vi "NewArray2.vi"(6 "Function":enum16{"Default", "Split to new"}(ring)=enum."Split to new", 7 "Map ref":refnum<vi>, 8 "error in (no error)":errorcluster, 11 "All Lines":T1) -> (0 "error out":errorcluster, 3 "output array":T1)   [LabVIEW 2014]
uses:
  Libraries/Map Data Folder/All-Lines.ctl
  Libraries/Map Data Folder/LineCluster.ctl
  Libraries/Map Data Folder/LineConnection.ctl
  Libraries/Map Data Folder/Map Data.lvlib
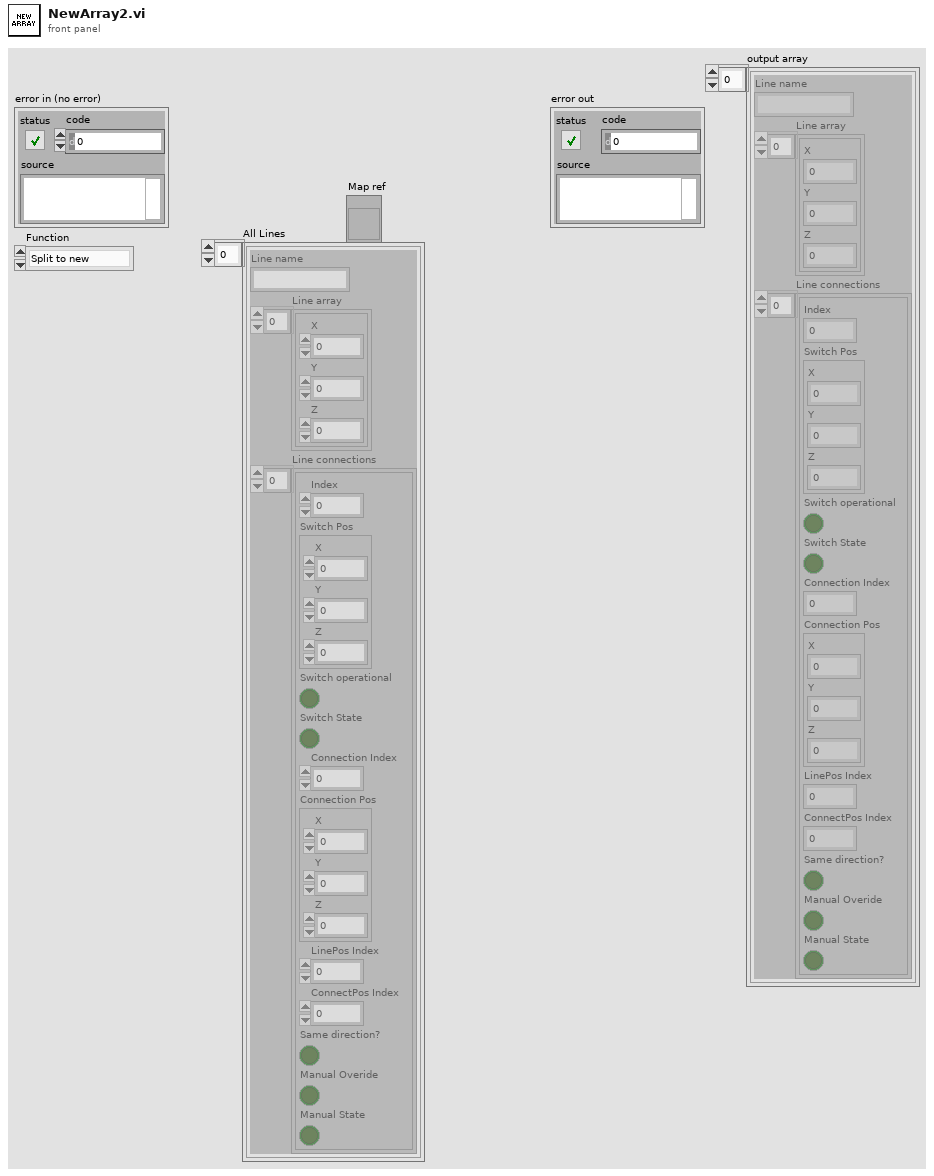
[diagram p1: front panel]
types:
  T1 = typedef "Map Data.lvlib/All-Lines.ctl" = T2[]
  T2 = typedef "Map Data.lvlib/LineCluster.ctl" = cluster{"Line name":string, "Line array":cluster{"X":dbl, "Y":dbl, "Z":dbl}[], "Line connections":T3[]}
  T3 = typedef "Map Data.lvlib/LineConnection.ctl" = cluster{"Index":i32, "Switch Pos":cluster{"X":dbl, "Y":dbl, "Z":dbl}, "Switch operational":bool, "Switch State":bool, "Connection Index":i32, "Connection Pos":cluster{"X":dbl, "Y":dbl, "Z":dbl}, "LinePos Index":i32, "ConnectPos Index":i32, "Same direction?":bool, "Manual Overide":bool, "Manual State":bool}
  T4 = typedef "LVCursorListTypeDef.ctl" = cluster{"Name":string, "Color":u32, "Style":u8, "Point Style":u8, "Name Visible":bool, "Allow Drag":bool, "Cursor Mode":u32, "Plot":i32, "Index":i32, "Position":cluster{"X":dbl, "Y":dbl}, "X Scale":u32, "Y Scale":u32, "Watch Plots":i32[], "Watch All Plots":bool, "Plot Area":i32, "Label Offset":cluster{"X":dbl, "Y":dbl}}[]
  T5 = cluster{"Name":string, "Color":u32, "Style":u8, "Point Style":u8, "Name Visible":bool, "Allow Drag":bool, "Cursor Mode":u32, "Plot":i32, "Index":i32, "Position":cluster{"X":dbl, "Y":dbl}, "X Scale":u32, "Y Scale":u32, "Watch Plots":i32[], "Watch All Plots":bool, "Plot Area":i32, "Label Offset":cluster{"X":dbl, "Y":dbl}}
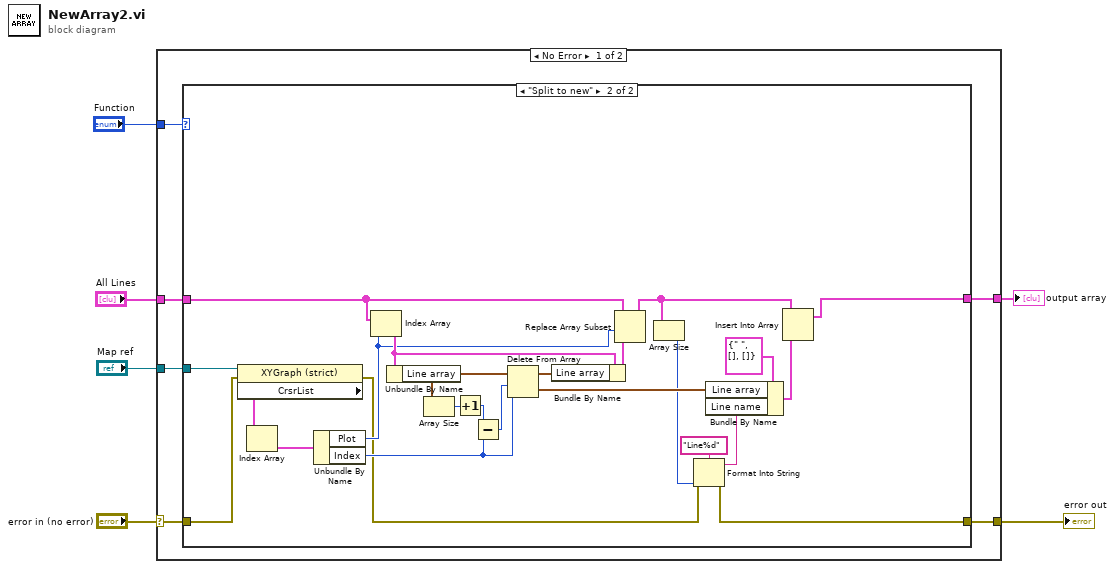
[diagram p0: block diagram]
diagram:
  n1 = case shown="No Error" "error in (no error)" {
    selector: "error in (no error)" -> [w10 w39]
    tunnel: "Map ref" -> [w12 _]
    tunnel: [w11 w39] -> w5
    tunnel: "Function" -> [w9 _]
    tunnel: "All Lines" -> [w8 w40]
    tunnel: [w7 w40] -> w1
    frame No Error {
      n2 = case shown="\"Split to new\"" w9 {
        tunnel: w12 -> [_ w36]
        tunnel: [w14 w15] -> w11
        tunnel: w10 -> [w14 w35]
        tunnel: w8 -> [w13 w25]
        tunnel: [w13 w17] -> w7
        frame "Default", Default {
        }
        frame "Split to new" {
          n3 = property on="Property Node" class="XYGraph (strict)"(reference=w36, error in=w35) -> (error out=w16:errorcluster, "CrsrList"=w38:T4)  [unwired: 1 out]
          n4 = Index Array(array=w38) -> (element=w37:T5)  [unwired: 1 in]
          n5 = Unbundle By Name(w37) -> ("Plot"=w26:i32, "Index"=w30:i32)
          n6 = Index Array(array=w25, index=w26) -> (element=w34:T2)
          n7 = Unbundle By Name(w34) -> ("Line array"=w32:cluster{"X":dbl, "Y":dbl, "Z":dbl}[])
          n8 = Array Size(array=w32) -> (size(s)=w31:i32)
          n9 = Increment(x=w31) -> (x+1=w28:i32)
          n10 = Subtract(x=w28, y=w30) -> (x-y=w29:i32)
          n11 = Delete From Array(array=w32, length=w29, index=w30) -> (deleted portion=w22:cluster{"X":dbl, "Y":dbl, "Z":dbl}[], array with subset deleted=w33:cluster{"X":dbl, "Y":dbl, "Z":dbl}[])
          n12 = Bundle By Name(cluster=w34, "Line array"=w33) -> (w27:T2)
          n13 = Replace Array Subset(array=w25, new element=w27, index=w26) -> (w21:T1)
          n14 = Array Size(array=w21) -> (size(s)=w20:i32)
          n15 = Format Into String(format string="Line%d", error in=w16, w20) -> (resulting string=w23:string, error out=w15:errorcluster)  [unwired: 1 in]
          n16 = Bundle By Name(cluster=T2 {"Line name"=" ", "Line array"=[], "Line connections"=[]} ("Line Cluster 2"), "Line array"=w22, "Line name"=w23) -> (w18:T2)
          n17 = Insert Into Array(array=w21, new element=w18) -> (w17:T1)  [unwired: 1 in]
        }
      }
    }
    frame Error {
    }
  }
  "error out" <- w5
  "output array" <- w1
